vi "Teleop.vi"(10 "Match Info":T3={"Autonomous Elapsed Seconds"=0.0, "TeleOp Elapsed Seconds"=0.0, "Disabled Elapsed Seconds"=0.0, "Visited Autonomous"=FALSE, "Visited TeleOp"=FALSE, "Visited Disabled"=FALSE, "Autonomous Settings"={"Autonomous Style"=enum."Independent", "VI Refnum"=refnum}}, 11 "Call Context":T4) -> ()   [LabVIEW 2013]
doc: "This VI is called for each TeleOp packet received from the DS where the robot is not disabled. It is often used to read from the joysticks and update I/O or to update setpoints for timed control loops. It should complete and return within 20 milliseconds or it may miss DS packets."
uses:
  <vilib>/Rock Robotics/WPI/DriverStation/WPI_DriverStationDerivedRobotMode.ctl
  <vilib>/Rock Robotics/WPI/DriverStation/WPI_DriverStationMatch Info.ctl
  <vilib>/Rock Robotics/WPI/DriverStation/WPI_DriverStationAllianceInfo.ctl
  <vilib>/Rock Robotics/WPI/DriverStation/WPI_DriverStationPositionInfo.ctl
  Robot Global Data.vi
  <vilib>/Rock Robotics/WPI/Joystick/WPI_JoystickGetSetRefNum.vi
panel:
  out "Position":T1
  out "Alliance":T2
  out "Analog 4 (V)":dbl
  out "Analog 3 (V)":dbl
  out "Analog 2 (V)":dbl
  out "Analog 1 (V)":dbl
  out "Driver Station Digital Input (1-8)":bool[](array[boolean])
  out "joy2_A1":dbl
  out "joy2_A2":dbl
  out "joy2_A3":dbl
  out "joy2_A4":dbl
  out "joy2_A5":dbl
  out "joy2_A6":dbl
  out "joy2_B1":bool
  out "joy2_B2":bool
  out "joy2_B3":bool
  out "joy2_B4":bool
  out "joy2_B6":bool
  out "joy2_B5":bool
  out "joy2_B7":bool
  out "joy2_B8":bool
  out "joy2_B9":bool
  out "joy2_B10":bool
  out "joy2_B11":bool
  out "joy2_B12":bool
  out "joy1_B12":bool
  out "joy1_B11":bool
  out "joy1_B10":bool
  out "joy1_B9":bool
  out "joy1_B8":bool
  out "joy1_B7":bool
  out "joy1_B6":bool
  out "joy1_B5":bool
  out "joy1_B4":bool
  out "joy1_B3":bool
  out "joy1_B2":bool
  out "joy1_B1":bool
  out "joy1_A6":dbl
  out "joy1_A5":dbl
  out "joy1_A4":dbl
  out "joy1_A3":dbl
  out "joy1_A2":dbl
  out "joy1_A1":dbl
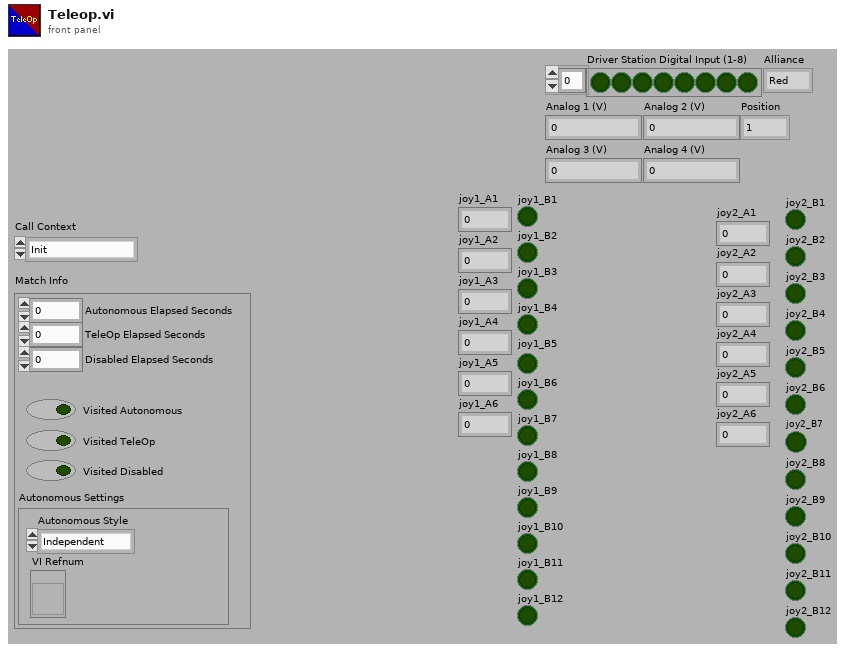
[diagram p1: front panel]
types:
  T1 = typedef "WPI_DriverStationPositionInfo.ctl" = enum16{"1", "2", "3"}
  T2 = typedef "WPI_DriverStationAllianceInfo.ctl" = enum16{"Red", "Blue", "Invalid"}
  T3 = typedef "WPI_DriverStationMatch Info.ctl" = cluster{"Autonomous Elapsed Seconds":dbl, "TeleOp Elapsed Seconds":dbl, "Disabled Elapsed Seconds":dbl, "Visited Autonomous":bool, "Visited TeleOp":bool, "Visited Disabled":bool, "Autonomous Settings":cluster{"Autonomous Style":enum16{"Iterative", "Independent"}, "VI Refnum":refnum<vi>}}
  T4 = typedef "WPI_DriverStationDerivedRobotMode.ctl" = enum16{"Init", "Execute", "Stop"}
  T5 = typedef "WPI_JoystickDevRef.ctl" = cluster{"Device":T6}
  T6 = typedef "WPI_JoystickDeviceEnum.ctl" = enum16{"USB 1", "USB 2", "USB 3", "USB 4", "Kinect 1", "Kinect 2"}
  T7 = typedef "WPI_JoystickButtonState.ctl" = cluster{"Button 1":bool, "Button 2":bool, "Button 3":bool, "Button 4":bool, "Button 5":bool, "Button 6":bool, "Button 7":bool, "Button 8":bool, "Button 9":bool, "Button 10":bool, "Button 11":bool, "Button 12":bool}
  T8 = cluster{"axis 1 (x)":dbl, "axis 2 (y)":dbl, "axis 3 (throttle)":dbl, "axis 4":dbl, "axis 5":dbl, "axis 6":dbl}
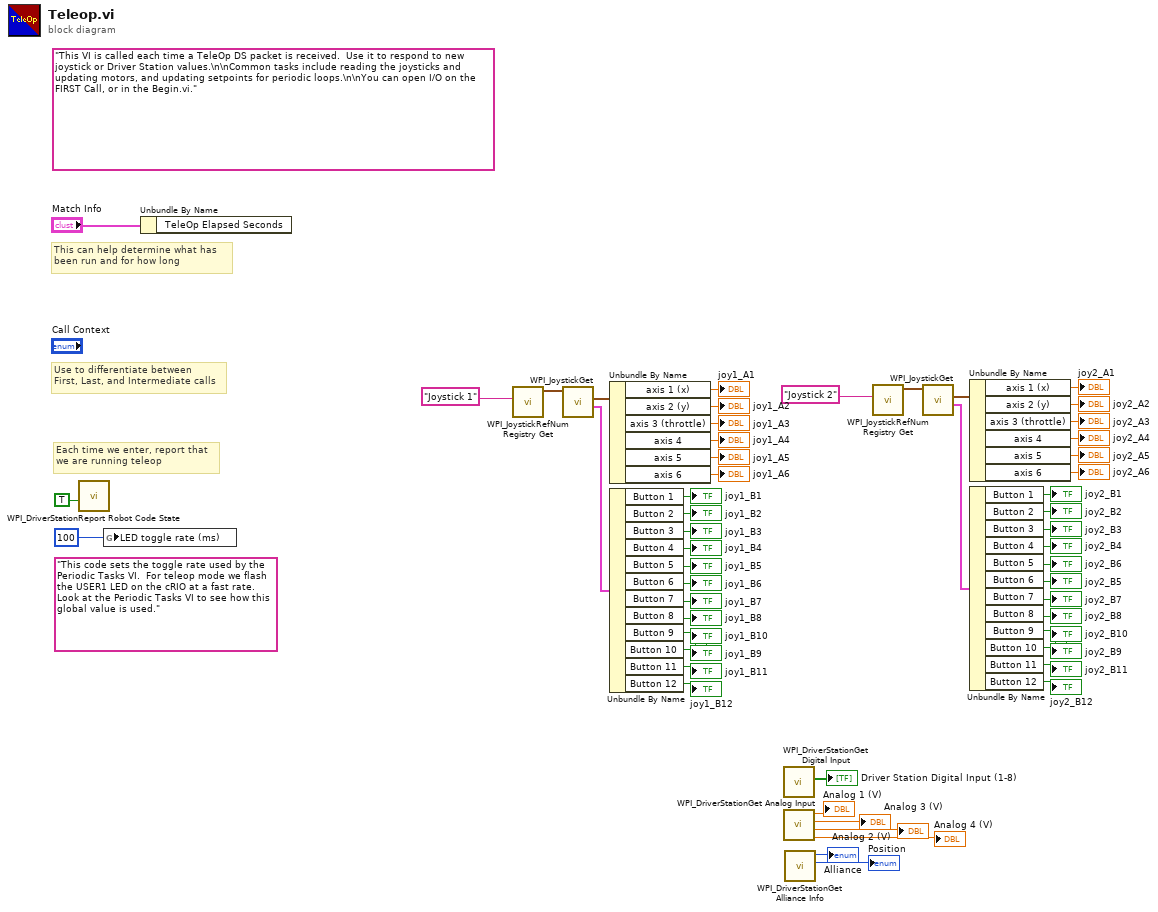
[diagram p0: block diagram]
diagram:
  (unwired) "This code sets the toggle rate used by the Periodic Tasks VI.  For teleop mode we flash the USER1 LED on the cRIO at a fast rate.  Look at the Periodic Tasks VI to see how this global value is used."
  (unwired) "This VI is called each time a TeleOp DS packet is received.  Use it to respond to new joystick or Driver Station values.\n\nCommon tasks include reading the joysticks and updating motors, and updating setpoints for periodic loops.\n\nYou can open I/O on the FIRST Call, or in the Begin.vi."
  # "Each time we enter, report that\nwe are running teleop"
  # "Use to differentiate between\nFirst, Last, and Intermediate calls"
  # "This can help determine what has\nbeen run and for how long"
  n1 = call <vilib>:"WPI_DriverStationReport Robot Code State.vi"("TeleOp"=TRUE ("Autonomous")) -> ()  [unwired: 10 in, 1 out]
  n2 = global write "Robot Global Data.vi" "LED toggle rate (ms)"(u32 100 ("LED ms toggle rate")) -> ()
  n3 = Unbundle By Name("Match Info") -> ()  [unwired: 1 out]
  n4 = call <vilib>:"WPI_JoystickRefNum Registry Get.vi"("refnum name"="Joystick 1") -> ("JoystickDevRef"=w52:T5)  [unwired: 1 in, 9 out]
  n5 = call <vilib>:"WPI_JoystickGet.vi"("JoystickDevRef"=w52) -> ("Buttons"=w42:T7, "Axes"=w49:T8)  [unwired: 1 in, 4 out]
  n6 = Unbundle By Name(w49) -> ("axis 1 (x)"=→"joy1_A1":dbl, "axis 2 (y)"=→"joy1_A2":dbl, "axis 3 (throttle)"=→"joy1_A3":dbl, "axis 4"=→"joy1_A4":dbl, "axis 5"=→"joy1_A5":dbl, "axis 6"=→"joy1_A6":dbl)
  n7 = Unbundle By Name(w42) -> ("Button 1"=→"joy1_B1":bool, "Button 2"=→"joy1_B2":bool, "Button 3"=→"joy1_B3":bool, "Button 4"=→"joy1_B4":bool, "Button 5"=→"joy1_B5":bool, "Button 6"=→"joy1_B6":bool, "Button 7"=→"joy1_B7":bool, "Button 8"=→"joy1_B8":bool, "Button 9"=→"joy1_B9":bool, "Button 10"=→"joy1_B10":bool, "Button 11"=→"joy1_B11":bool, "Button 12"=→"joy1_B12":bool)
  n8 = call <vilib>:"WPI_DriverStationGet Digital Input.vi"() -> ("Driver Station Digital Input (1-8)"=→"Driver Station Digital Input (1-8)":bool[])  [unwired: 11 in]
  n9 = call <vilib>:"WPI_DriverStationGet Analog Input.vi"() -> ("Analog 4 (V)"=→"Analog 4 (V)":dbl, "Analog 3 (V)"=→"Analog 3 (V)":dbl, "Analog 2 (V)"=→"Analog 2 (V)":dbl, "Analog 1 (V)"=→"Analog 1 (V)":dbl)  [unwired: 8 in]
  n10 = call <vilib>:"WPI_DriverStationGet Alliance Info.vi"() -> ("Position"=→"Position":T1, "Alliance"=→"Alliance":T2)  [unwired: 10 in]
  n11 = call <vilib>:"WPI_JoystickRefNum Registry Get.vi"("refnum name"="Joystick 2") -> ("JoystickDevRef"=w9:T5)  [unwired: 1 in, 9 out]
  n12 = call <vilib>:"WPI_JoystickGet.vi"("JoystickDevRef"=w9) -> ("Buttons"=w17:T7, "Axes"=w10:T8)  [unwired: 1 in, 4 out]
  n13 = Unbundle By Name(w10) -> ("axis 1 (x)"=→"joy2_A1":dbl, "axis 2 (y)"=→"joy2_A2":dbl, "axis 3 (throttle)"=→"joy2_A3":dbl, "axis 4"=→"joy2_A4":dbl, "axis 5"=→"joy2_A5":dbl, "axis 6"=→"joy2_A6":dbl)
  n14 = Unbundle By Name(w17) -> ("Button 1"=→"joy2_B1":bool, "Button 2"=→"joy2_B2":bool, "Button 3"=→"joy2_B3":bool, "Button 4"=→"joy2_B4":bool, "Button 5"=→"joy2_B6":bool, "Button 6"=→"joy2_B5":bool, "Button 7"=→"joy2_B7":bool, "Button 8"=→"joy2_B8":bool, "Button 9"=→"joy2_B9":bool, "Button 10"=→"joy2_B10":bool, "Button 11"=→"joy2_B11":bool, "Button 12"=→"joy2_B12":bool)
